vi "Set API Key.vi"(8 "Error In":errorcluster, 10 "API Key":string, 11 "Open Weather Session In":refnum<class "Open Weather Session.lvclass">) -> (0 "Error Out":errorcluster, 3 "Open Weather Session Out":refnum<class "Open Weather Session.lvclass">)   [LabVIEW 2019, in "Open Weather Session.lvclass"]
uses:
  Open Weather Session.lvclass
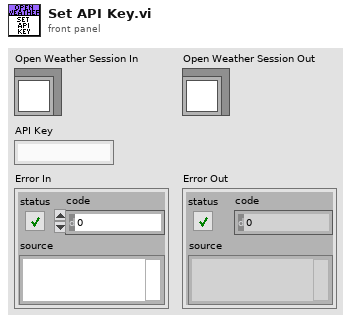
[diagram p1: front panel]
types:
  T1 = typedef "Open Weather Session.lvclass/Data.ctl" = cluster{"API Key":string, "REST Client":refnum<class "REST Client.lvclass">}
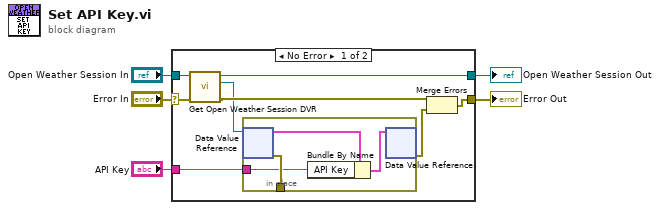
[diagram p0: block diagram]
diagram:
  n1 = case shown="No Error" "Error In" {
    selector: "Error In" -> [w9 w18]
    tunnel: [w12 w18] -> w2
    tunnel: [w8 w19] -> w5
    tunnel: "Open Weather Session In" -> [w10 w19]
    tunnel: "API Key" -> [w11 _]
    frame No Error {
      n2 = call "Get Open Weather Session DVR.vi"("Error In"=w9, "Open Weather Session In"=w10) -> ("Error Out"=w7:errorcluster, "DVR"=w6:refnum<data-value>, "Open Weather Session Out"=w8:refnum<class "Open Weather Session.lvclass">)  [unwired: 7 in]
      n3 = in-place {
        in-place-border: [w17] -> _
        in-place-border: w11 -> [w14]
        n4 = in-place-dvr #1(w6) -> (w16:T1, w17:errorcluster)
        n5 = Bundle By Name(cluster=w16, "API Key"=w14) -> (w15:T1)
        n6 = in-place-dvr #1(w15) -> (w13:errorcluster)  [unwired: 1 out]
      }
      n7 = Merge Errors(w7, w13) -> (w12:errorcluster)
    }
    frame Error {
    }
  }
  "Open Weather Session Out" <- w5
  "Error Out" <- w2
